vi "Benchmark Convert String Type - Random Scalars.vi"(8 "iterations (1)":i32=1, 9 "dst byte order":T1(ring)=enum."native, host order", 10 "src byte order":T1(ring), 11 "channel count":i32=10000 format="%#.3p") -> (0 "error out":errorcluster, 3 "duration":dbl format="%.0ps")   [LabVIEW 2017]
uses:
  Classes/Buffer Converter/Convert String Type Subset.vi
  Shared/VIs/Sizeof 1D.vi
  Shared/VIs/Sizeof.vi
  Classes/Buffer Converter/Buffer Converter.lvclass
panel:
  out "dst buffer size":u64 format="%.0pB"
  out "src buffer size":u64 format="%.0pB"
  out "src buffer":string
  out "dst buffer":string
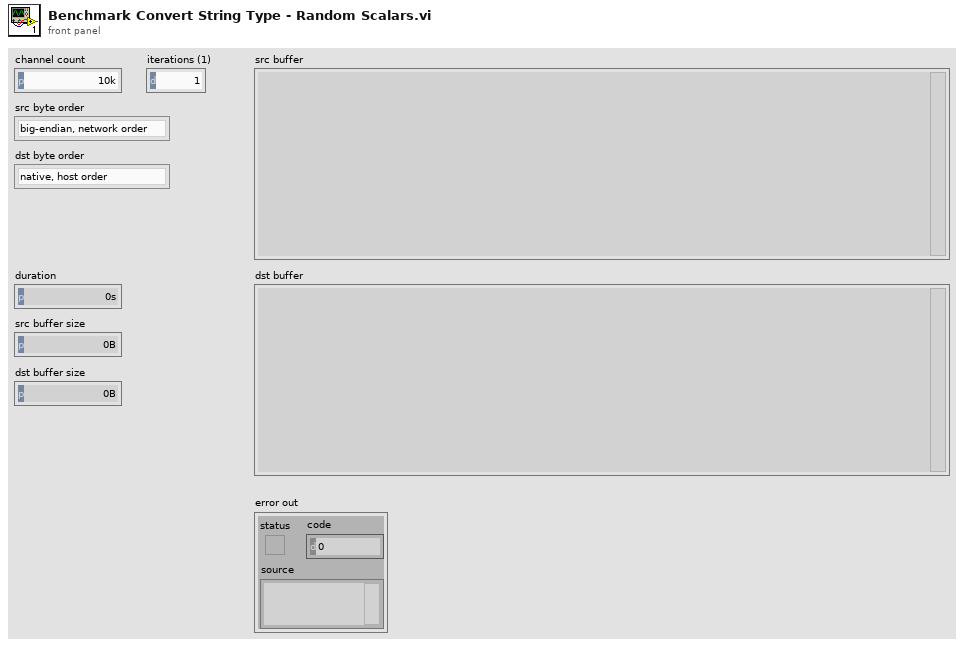
[diagram p1: front panel]
types:
  T1 = enum16{"big-endian, network order", "native, host order", "little-endian"}
  T2 = typedef "DSF Core.lvlib/Buffer Converter.lvclass/Type Conversion.ctl" = cluster{"unconverted descriptor":T3, "converted descriptor":T3, "channel count":u64}
  T3 = typedef "DSF Core.lvlib/Buffer.lvclass/Channel Descriptor.ctl" = cluster{"buffer offset":u64, "data type":T4}
  T4 = typedef "DSF Core.lvlib/DSF Data Type.ctl" = enum8{"Bool", "SGL", "DBL", "I8", "I16", "I32", "I64", "U8", "U16", "U32", "U64"}
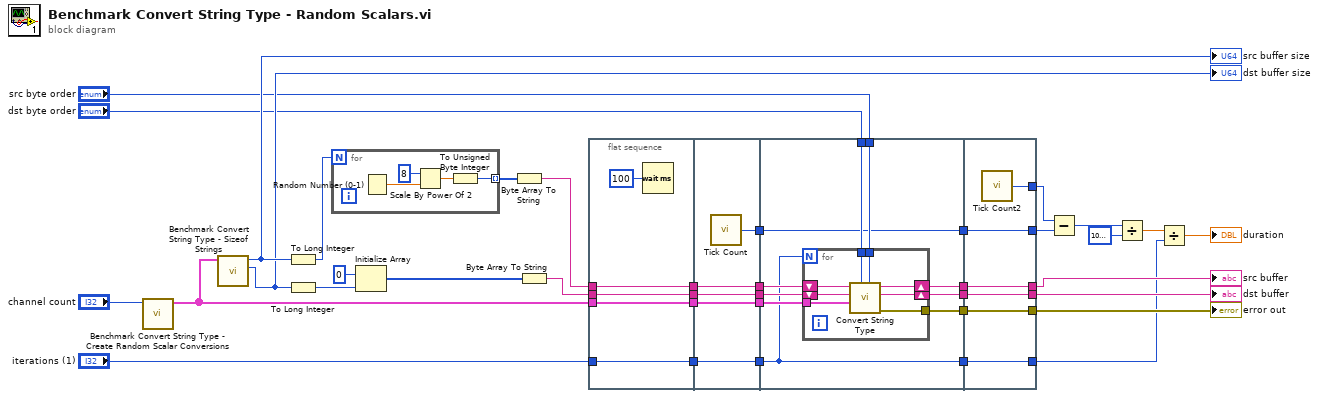
[diagram p0: block diagram]
diagram:
  n1 = call "Benchmark Convert String Type - Create Random Scalar Conversions.vi"("channel count"="channel count") -> ("conversions"=w38:T2[])  [unwired: 10 in]
  n2 = call "Benchmark Convert String Type - Sizeof Strings.vi"("conversions"=w38) -> ("converted string size"=w35:u64, "unconverted string size"=w37:u64)  [unwired: 9 in]
  "src buffer size" <- w37
  "dst buffer size" <- w35
  n3 = To Long Integer(number=w37) -> (32bit integer=w10:i32)
  n4 = To Long Integer(number=w35) -> (32bit integer=w34:i32)
  n5 = for {
    N: w10 -> [_]
    tunnel: [w39] -> w9 mode=indexing
    n6 = Random Number (0-1)() -> (number: 0 to 1=w41:dbl)
    n7 = Scale By Power Of 2(n=i16 8, x=w41) -> (x*2^n=w40:dbl)
    n8 = To Unsigned Byte Integer(number=w40) -> (unsigned 8bit integer=w39:u8)
  }
  n9 = Initialize Array(u8 0 ("element"), w34) -> (w33:u8[])
  n10 = Byte Array To String(unsigned byte array=w9) -> (string=w32:string)
  n11 = Byte Array To String(unsigned byte array=w33) -> (string=w8:string)
  n12 = flat-sequence {
    tunnel: w32 -> [w45]
    tunnel: w8 -> [w46]
    tunnel: w38 -> [w47]
    tunnel: [w47] -> w19
    tunnel: [w46] -> w18
    tunnel: [w45] -> w17
    tunnel: "iterations (1)" -> [w43]
    tunnel: [w43] -> w6
    tunnel: [w52] -> w22
    tunnel: [w51] -> w21
    tunnel: [w50] -> w20
    tunnel: w19 -> [w52]
    tunnel: w18 -> [w51]
    tunnel: w17 -> [w50]
    tunnel: [w49] -> w16
    tunnel: w6 -> [w48]
    tunnel: [w48] -> w5
    tunnel: "dst byte order" -> [w59]
    tunnel: "src byte order" -> [w58]
    tunnel: [w57] -> w25
    tunnel: [w56] -> w24
    tunnel: [w55] -> w23
    tunnel: w22 -> [w62]
    tunnel: w21 -> [w61]
    tunnel: w20 -> [w60]
    tunnel: w16 -> [w54]
    tunnel: [w54] -> w15
    tunnel: w5 -> [w53]
    tunnel: [w53] -> w4
    tunnel: [w74] -> w27
    tunnel: [w75] -> w28
    tunnel: [w76] -> w29
    tunnel: w25 -> [w76]
    tunnel: w24 -> [w75]
    tunnel: w23 -> [w74]
    tunnel: [w73] -> w13
    tunnel: w15 -> [w72]
    tunnel: [w72] -> w14
    tunnel: w4 -> [w71]
    tunnel: [w71] -> w3
    frame #0 {
      n13 = Wait (ms)(milliseconds to wait=u32 100) -> ()  [unwired: 1 out]
    }
    frame #1 {
      n14 = call "Tick Count"() -> ("Tick Count(uSec)"=w49:u32)
    }
    frame #2 {
      n15 = for {
        N: w53 -> [_]
        tunnel: w62 -> [w70]
        tunnel: w59 -> [w67]
        tunnel: w58 -> [w66]
        tunnel: [w65] -> w57
        shift-right: [w64] -> w56
        shift-left: w61 -> [w69]
        shift-right: [w63] -> w55
        shift-left: w60 -> [w68]
        n16 = call "Convert String Type.vi"("src byte order"=w66, "dst byte order"=w67, "conversions"=w70, "dst buffer in"=w69, "src buffer in"=w68) -> ("error out"=w65:errorcluster, "dst buffer out"=w64:string, "src buffer out"=w63:string)  [unwired: 4 in]
      }
    }
    frame #3 {
      n17 = call "Tick Count2"() -> ("Tick Count(uSec)"=w73:u32)
    }
  }
  n18 = Subtract(x=w13, y=w14) -> (x-y=w12:u32)
  n19 = Divide(x=w12, y=u32 1000000) -> (x/y=w2:dbl)
  n20 = Divide(x=w2, y=w3) -> (x/y=→"duration":dbl)
  "error out" <- w29
  "dst buffer" <- w28
  "src buffer" <- w27
